vi "Run_Init Core.vi"(0 "Array Functions in":refnum<class "Array Functions.lvclass">, 11 "error in (no error)":errorcluster) -> (4 "Array Functions out":refnum<class "Array Functions.lvclass">, 15 "error out":errorcluster)   [LabVIEW 2019, in "Array Functions.lvclass"]
uses:
  Array Functions.lvclass
  C:/Users/Patrick/Documents/GitHub/LabVIEW-Script-Language/source code/LSL components/functions/functionsbase/functionbase.lvclass
  functionsbase/functionbase.lvclass
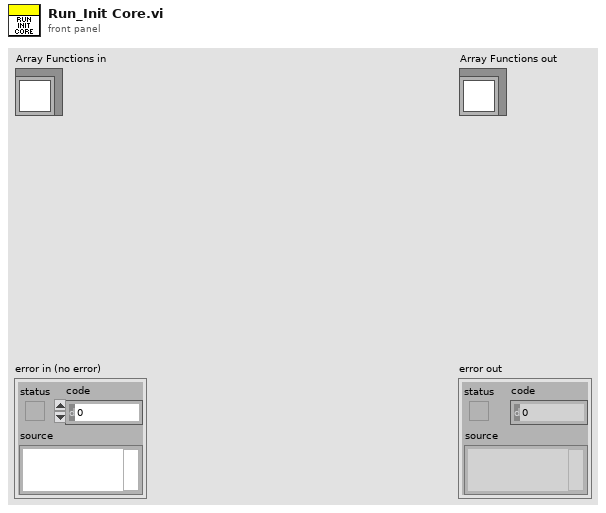
[diagram p1: front panel]
types:
  T1 = typedef "Valuetype.ctl" = enum16{"Value", "Variable", "Function"}
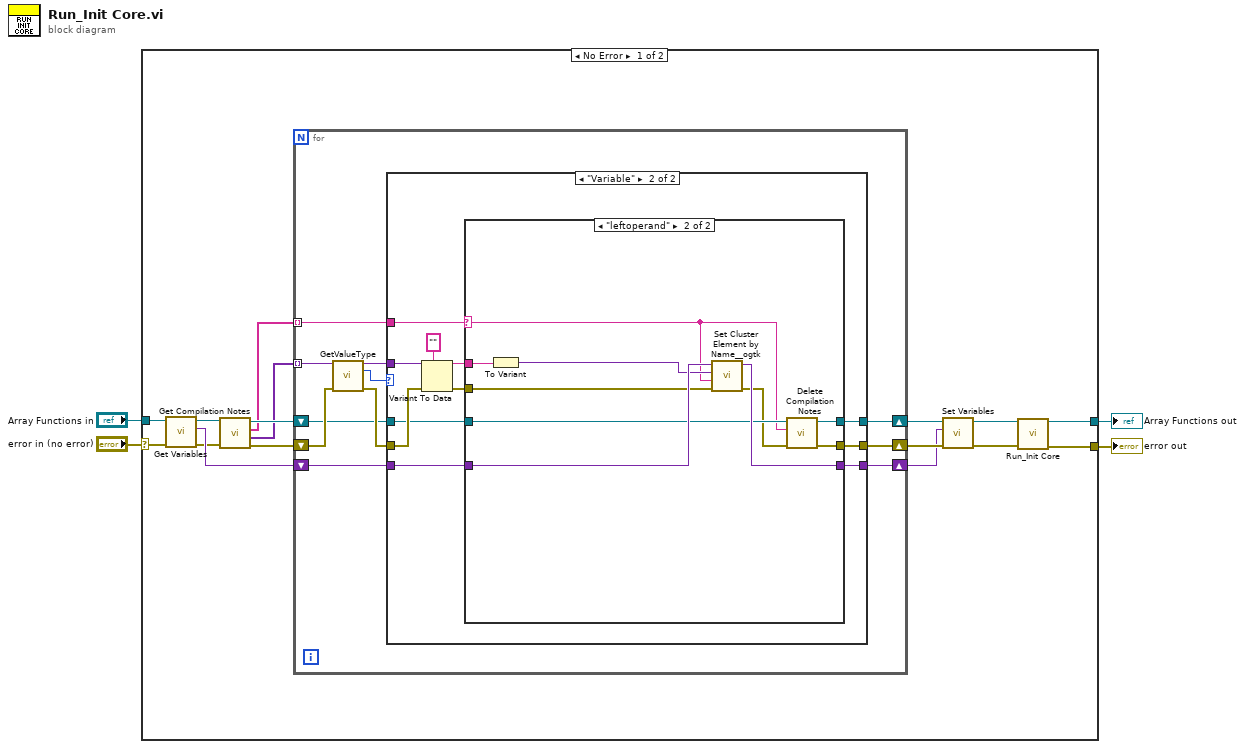
[diagram p0: block diagram]
diagram:
  n1 = case shown="No Error" "error in (no error)" {
    selector: "error in (no error)" -> [w20 w60]
    tunnel: [w5 w60] -> w1
    tunnel: [w7 w59] -> w2
    tunnel: "Array Functions in" -> [w19 w59]
    frame No Error {
      n2 = call-dynamic "Get Variables.vi"("error in (no error)"=w20, "Message Popup in"=w19) -> ("error out"=w14:errorcluster, "Variables"=w18:variant, "Message Popup out"=w13:refnum<class "Array Functions.lvclass">)  [unwired: 7 in]
      n3 = call "Get Compilation Notes.vi"("error in (no error)"=w14, "functionbase in"=w13) -> ("error out"=w12:errorcluster, "note"=w10:variant[], "note Key"=w9:string[], "functionbase out"=w11:refnum<class "Array Functions.lvclass">)  [unwired: 6 in]
      n4 = for {
        shift-right: [w21] -> w17
        shift-left: w11 -> [w22]
        shift-right: [w30] -> w15
        shift-left: w18 -> [w31]
        shift-right: [w29] -> w16
        shift-left: w12 -> [w27]
        tunnel: w10 -> [w28] mode=indexing
        tunnel: w9 -> [w26] mode=indexing
        n5 = call "GetValueType.vi"("variant"=w28, "error in"=w27) -> ("variant out"=w24:variant, "Value Type"=w25:T1, "error out"=w23:errorcluster)  [unwired: 11 in]
        n6 = case shown="\"Variable\"" w25 {
          tunnel: w24 -> [_ w44]
          tunnel: [w34 w39] -> w30
          tunnel: w31 -> [w34 w40]
          tunnel: [w33 w38] -> w29
          tunnel: w23 -> [w33 w45]
          tunnel: w26 -> [_ w37]
          tunnel: w22 -> [w32 w36]
          tunnel: [w32 w35] -> w21
          frame Default {
          }
          frame "Variable" {
            n7 = Variant To Data(error in=w45, type="", Variant=w44) -> (data=w41:string, error out=w42:errorcluster)
            n8 = case shown="\"leftoperand\"" w37 {
              selector: w37 -> [_ w49]
              tunnel: w42 -> [w47 w56]
              tunnel: w41 -> [_ w55]
              tunnel: w40 -> [w48 w58]
              tunnel: [w48 w57] -> w39
              tunnel: [w47 w50] -> w38
              tunnel: w36 -> [w46 w53]
              tunnel: [w46 w52] -> w35
              frame Default {
              }
              frame "leftoperand" {
                n9 = To Variant(anything=w55) -> (Variant=w54:variant)
                n10 = call <userlib>:"Set Cluster Element by Name__ogtk.vi"("error in (no error)"=w56, "Element Name (\"\": New Element Data Name)"=w49, "New Element Value"=w54, "Cluster"=w58) -> ("error out"=w51:errorcluster, "VCluster out"=w57:variant)  [unwired: 5 in, 1 out]
                n11 = call "Delete Compilation Notes.vi"("error in (no error)"=w51, "note key"=w49, "functionbase in"=w53) -> ("error out"=w50:errorcluster, "functionbase out"=w52:refnum<class "Array Functions.lvclass">)  [unwired: 7 in]
              }
            }
          }
        }
      }
      n12 = call-dynamic "Set Variables.vi"("error in (no error)"=w16, "Variables"=w15, "Message Popup in"=w17) -> ("error out"=w6:errorcluster, "Message Popup out"=w8:refnum<class "Array Functions.lvclass">)  [unwired: 7 in]
      n13 = call-parent "Run_Init Core.vi"("functionbase in"=w8, "error in (no error)"=w6) -> ("functionbase out"=w7:refnum<class "Array Functions.lvclass">, "error out"=w5:errorcluster)  [unwired: 12 in]
    }
    frame Error {
    }
  }
  "error out" <- w1
  "Array Functions out" <- w2
